vi "eFGV - Stop HMI.vi"(6 "Action":T1, 8 "Error In":errorcluster, 11 "Stop HMI? In":bool) -> (0 "Error Out":errorcluster, 2 "Event Stop HMI":refnum<user-event>, 3 "Stop HMI? Out":bool)   [LabVIEW 2020]
uses:
  Control/State - eFGV.ctl
  <vilib>/event_ctls.llb/usereventprio.ctl
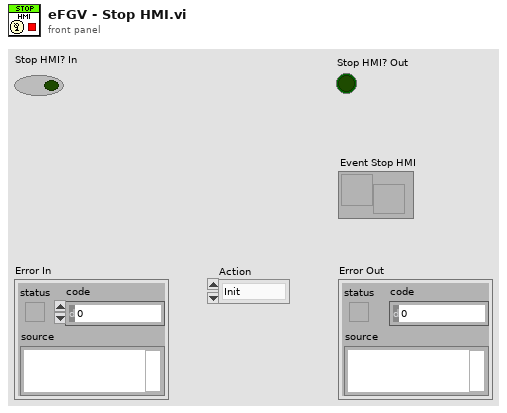
[diagram p1: front panel]
types:
  T1 = typedef "State - eFGV.ctl" = enum16{"Init", "Read", "Write", "Exit"}
  T2 = typedef "usereventprio.ctl" = enum32{"high priority", "normal priority"}
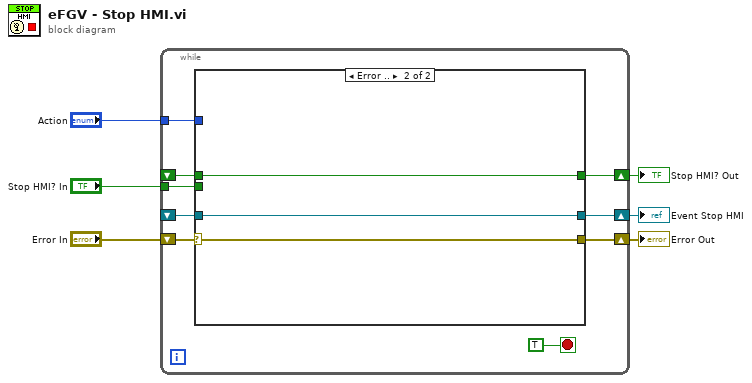
[diagram p0: block diagram]
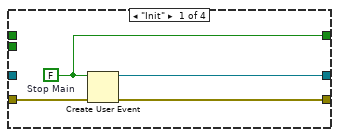
[diagram p3: hidden frame]
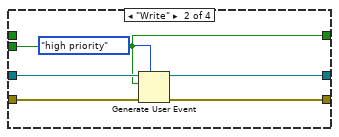
[diagram p4: hidden frame]
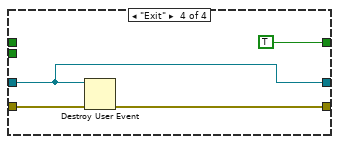
[diagram p5: hidden frame]
diagram:
  n1 = while {
    tunnel: "Action" -> [w12]
    shift-right: [w15] -> w6
    shift-left: "Error In" -> [w14]
    shift-right: [w11] -> w1
    shift-left: _ -> [w10]
    tunnel: "Stop HMI? In" -> [w9]
    shift-right: [w8] -> w2
    shift-left: _ -> [w7]
    stop <- TRUE stop-if-true
    n2 = case shown="Error .." w14 {
      selector: w14 -> [w22 w43]
      tunnel: [w23 w43] -> w15
      tunnel: w12 -> [w21 _]
      tunnel: [w20 w41] -> w11
      tunnel: w10 -> [w19 w41]
      tunnel: w9 -> [w18 _]
      tunnel: [w17 w42] -> w8
      tunnel: w7 -> [w16 w42]
      frame No Error {
        n3 = case shown="\"Read\"" w21 {
          tunnel: w22 -> [w27 w33 w36 w40]
          tunnel: [w26 w32 w36 w39] -> w23
          tunnel: [w25 w29 w35 w37] -> w20
          tunnel: w19 -> [_ w31 w35 w37]
          tunnel: w18 -> [_ w30 _ _]
          tunnel: [w24 w30 w34 TRUE ("Stop?")] -> w17
          tunnel: w16 -> [_ _ w34 _]
          frame "Init" {
            w24 = FALSE  # Stop Main
            n4 = Create User Event(user event datatype=w24, error in=w27) -> (user event=w25:refnum<user-event>, error out=w26:errorcluster)
          }
          frame "Write" {
            n5 = Generate User Event(priority (normal)=usereventprio."high priority", user event=w31, event data cluster=w30, error in=w33) -> (user event out=w29:refnum<user-event>, error out=w32:errorcluster)
          }
          frame "Read" {
          }
          frame "Exit" {
            n6 = Destroy User Event(user event=w37, error in=w40) -> (error out=w39:errorcluster)
          }
        }
      }
      frame Error {
      }
    }
  }
  "Error Out" <- w6
  "Stop HMI? Out" <- w2
  "Event Stop HMI" <- w1
